vi "Compile Digital Pattern Gen 1.3 Data.vi"(7 "RIO Address":string, 8 "error in (no error)":errorcluster, 11 "Device Item Ref in":T3 format="%.0x") -> (0 "error out":errorcluster, 1 "bitfile names":string[](array[string]), 2 "Digital Pattern Gens":T1[](array[typedef]), 3 "Device Item Ref out":T3 format="%.0x")   [LabVIEW 2017, in "Engine Simulation Toolkit System Explorer.lvlib"]
uses:
  Engine Simulation Toolkit System Explorer.lvlib
  <vilib>/NI Veristand/Custom Device API/Custom Device Item Ref.ctl
  Shared/1.3 Digital Pattern Gen Engine Data.ctl
  Shared/1.3 Digital Pattern Gen FIFO Idxs.ctl
  Digital Pattern Find Events Enum.ctl
  Shared/Constants and GUIDs.vi
  <vilib>/NI Veristand/Custom Device Tools/Custom Device Utility Library/NI VeriStand - Search for Item by GUID.vi
  <vilib>/NI Veristand/Custom Device Tools/Custom Device Utility Library/Custom Device Utility Library.lvlib
  Shared/Engine Simulation Toolkit Shared.lvlib
  <vilib>/NI Veristand/Custom Device API/Custom Device API.lvlib
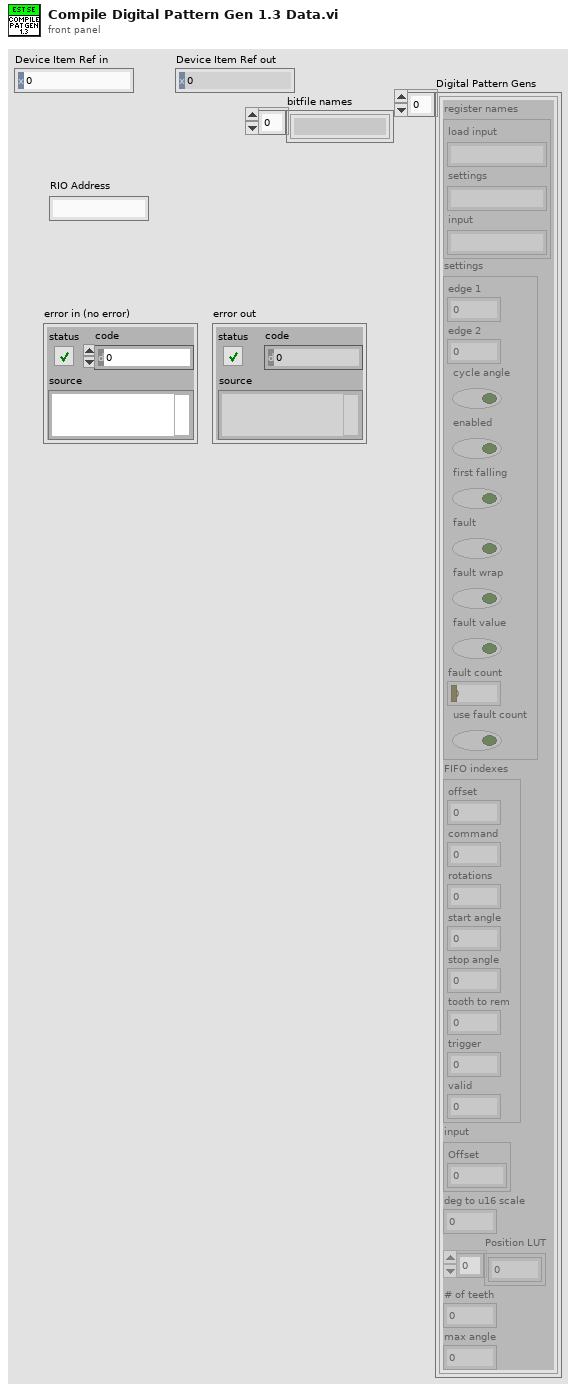
[diagram p1: front panel]
types:
  T1 = typedef "Engine Simulation Toolkit Shared.lvlib/1.3 Digital Pattern Gen Engine Data.ctl" = cluster{"register names":cluster{"load input":string, "settings":string, "input":string}, "settings":cluster{"edge 1":u16, "edge 2":u16, "cycle angle":bool, "enabled":bool, "first falling":bool, "fault":bool, "fault wrap":bool, "fault value":bool, "fault count":fxp<+,4,4>, "use fault count":bool}, "FIFO indexes":T2, "input":cluster{"Offset":i16}, "deg to u16 scale":dbl, "Position LUT":u16[], "# of teeth":i16, "max angle":dbl}
  T2 = typedef "Engine Simulation Toolkit Shared.lvlib/1.3 Digital Pattern Gen FIFO Idxs.ctl" = cluster{"offset":i32, "command":i32, "rotations":i32, "start angle":i32, "stop angle":i32, "tooth to rem":i32, "trigger":i32, "valid":i32}
  T3 = typedef "Custom Device API.lvlib/Custom Device Item Ref.ctl" = u64
  T4 = typedef "Engine Simulation Toolkit Shared.lvlib/Channel.ctl" = cluster{"Name":string, "Units":string, "Default":dbl, "Description":string, "Scalable":bool}
  T5 = typedef "Engine Simulation Toolkit System Explorer.lvlib/Digital Pattern.ctl" = cluster{"Name":string, "Base":T6, "Remove":T7[], "Add":T8[], "FPGA Resource":string}
  T6 = typedef "Engine Simulation Toolkit System Explorer.lvlib/Digital Pattern Base.ctl" = cluster{"Length":dbl, "Teeth":u16, "Width":dbl, "Offset":dbl}
  T7 = typedef "Engine Simulation Toolkit System Explorer.lvlib/Digital Pattern Remove Edge.ctl" = cluster{"Tooth":u16, "Edge":bool}
  T8 = typedef "Engine Simulation Toolkit System Explorer.lvlib/Digital Pattern Add Pulse.ctl" = cluster{"Tooth":u16, "Offset":dbl, "Width":dbl}
  T9 = typedef "Engine Simulation Toolkit System Explorer.lvlib/Digital Pattern Find Events Enum.ctl" = enum16{"Rising Edge", "Falling Edge", "Any Edge", "Center Tooth", "Center Gap"}
  T10 = typedef "Engine Simulation Toolkit System Explorer.lvlib/Digital Pattern Expanded.ctl" = cluster{"X":dbl[], "Y":dbl[]}
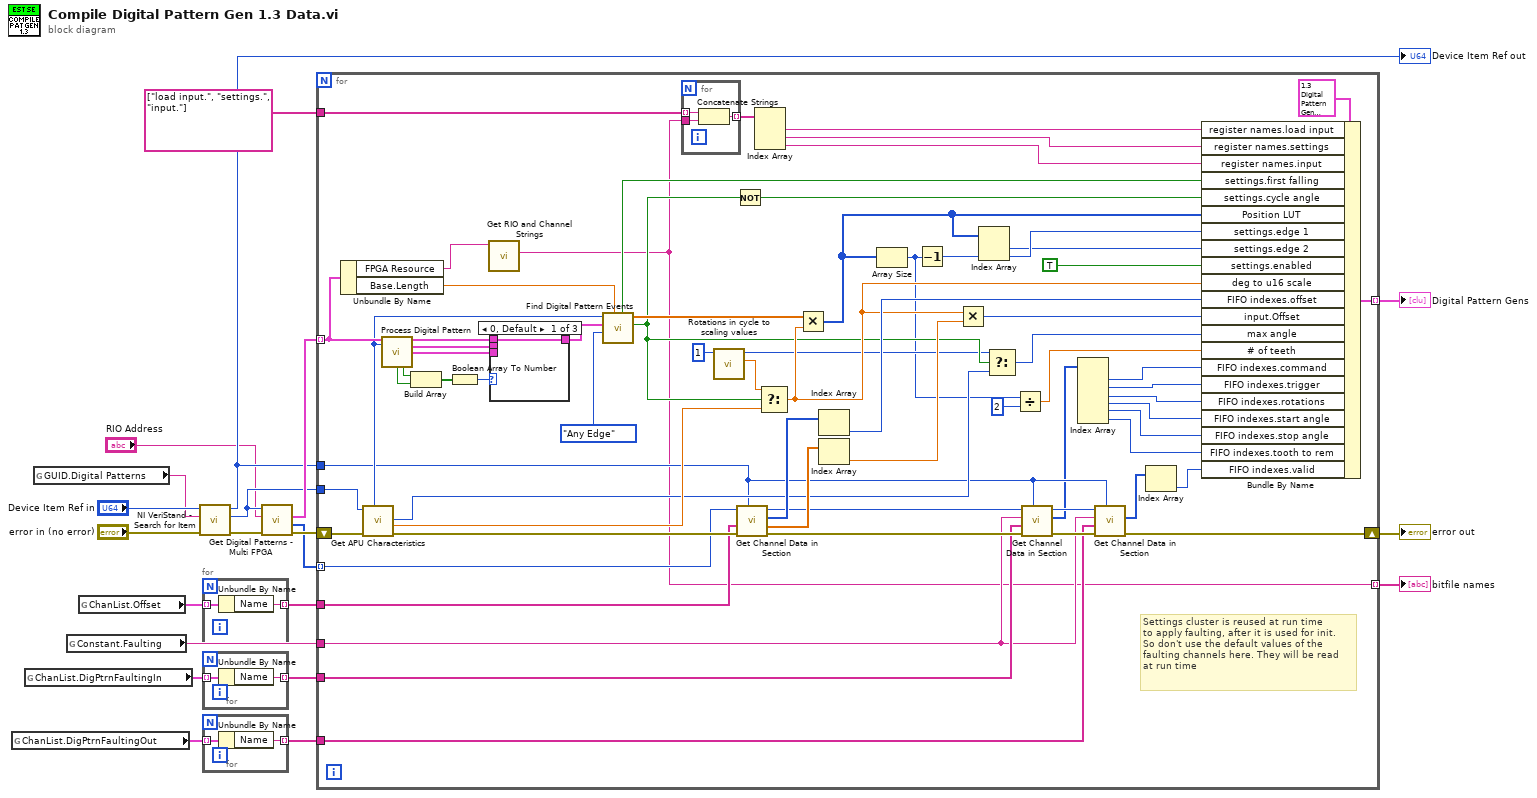
[diagram p0: block diagram]
diagram:
  n1 = global read "Constants and GUIDs.vi" "ChanList.DigPtrnFaultingOut"() -> (w5:T4[])
  n2 = global read "Constants and GUIDs.vi" "ChanList.DigPtrnFaultingIn"() -> (w6:T4[])
  n3 = global read "Constants and GUIDs.vi" "GUID.Digital Patterns"() -> (w19:string)
  n4 = global read "Constants and GUIDs.vi" "Constant.Faulting"() -> (w4:string)
  n5 = global read "Constants and GUIDs.vi" "ChanList.Offset"() -> (w8:T4[])
  n6 = call-poly <vilib>:"NI VeriStand - Search for Item.vi"("error in"="error in (no error)", "Item GUID"=w19, "Section Ref in"="Device Item Ref in") -> ("error out"=w18:errorcluster, "Item Ref"=w10:T3, "Section Ref out"=w11:T3)  [unwired: 5 in, 1 out]
  "Device Item Ref out" <- w11
  n7 = for {
    tunnel: [w23] -> w7 mode=indexing
    tunnel: w8 -> [w22] mode=indexing
    n8 = Unbundle By Name(w22) -> ("Name"=w23:string)
  }
  n9 = for {
    tunnel: [w25] -> w3 mode=indexing
    tunnel: w6 -> [w24] mode=indexing
    n10 = Unbundle By Name(w24) -> ("Name"=w25:string)
  }
  n11 = for {
    tunnel: [w27] -> w2 mode=indexing
    tunnel: w5 -> [w26] mode=indexing
    n12 = Unbundle By Name(w26) -> ("Name"=w27:string)
  }
  n13 = call "Get Digital Patterns - Multi FPGA.vi"("error in (no error)"=w18, "RIO Address"="RIO Address", "Item Ref in"=w10) -> ("error out"=w13:errorcluster, "references"=w9:T3[], "Patterns"=w12:T5[])  [unwired: 6 in]
  n14 = for {
    shift-right: [w30] -> w16
    shift-left: w13 -> [w87]
    tunnel: w12 -> [w85] mode=indexing
    tunnel: string[] ["load input.", "settings.", "input."] -> [w95]
    tunnel: [w90] -> w15 mode=indexing
    tunnel: [w28] -> w14 mode=indexing
    tunnel: w11 -> [w40]
    tunnel: w10 -> [w86]
    tunnel: w9 -> [w74] mode=indexing
    tunnel: w7 -> [w73]
    tunnel: w4 -> [w42]
    tunnel: w3 -> [w43]
    tunnel: w2 -> [w41]
    # "Settings cluster is reused at run time\nto apply faulting, after it is used for init.\nSo don't use the default values of the\nfaulting channels here. They will be read\nat run time"
    n15 = Unbundle By Name(w85) -> ("FPGA Resource"=w29:string, "Base.Length"=w83:dbl)
    n16 = call "Get APU Characteristics.vi"("error in (no error)"=w87, "Item Ref in"=w86) -> ("error out"=w81:errorcluster, "angle to u16 scale factor"=w57:dbl, "total angle span (degrees)"=w52:u16, "rotations"=w84:u16)  [unwired: 3 in, 3 out]
    n17 = call "Process Digital Pattern.vi"("EPT Pattern"=w85, "Rotations"=w84) -> ("Base"=w61:T10, 6:"Reduced"=w60:T10, 8:"Final"=w59:T10, 13:"Final"=w64:bool, 14:"Reduced"=w65:bool)  [unwired: 7 in, 2 out]
    n18 = Build Array(w65, w64) -> (w63:bool[])
    n19 = Boolean Array To Number(Boolean array=w63) -> (number=w62:u32)
    n20 = call "Get RIO and Channel Strings.vi"("rio/channel"=w29) -> ("channel"=w28:string)  [unwired: 9 in, 1 out]
    n21 = case shown="0, Default" w62 {
      tunnel: w61 -> [w96 _ _]
      tunnel: w60 -> [_ w97 _]
      tunnel: w59 -> [_ _ w98]
      tunnel: [w96 w97 w98] -> w58
      frame 0, Default {
      }
      frame 1 {
      }
      frame 2, 3 {
      }
    }
    n22 = call "Find Digital Pattern Events.vi"("Base.length"=w83, "Event"=Digital_Pattern_Find_Events_Enum."Any Edge", "Pattern"=w58, "Rotations"=w84) -> ("crank angle"=w54:bool, "Locations"=w80:dbl[], "first falling"=w55:bool)  [unwired: 5 in]
    n23 = for {
      tunnel: w28 -> [w101]
      tunnel: w95 -> [w100] mode=indexing
      tunnel: [w99] -> w93 mode=indexing
      n24 = Concatenate Strings(w100, w101) -> (w99:string)
    }
    n25 = call "Rotations in cycle to scaling values.vi"("rotations in a cycle"=u16 1) -> ("angle to u16 scale factor"=w56:dbl, "total angle span (degrees)"=w53:u16)  [unwired: 8 in, 1 out]
    n26 = Not(x=w54) -> (.not. x?=w66:bool)
    n27 = call "Get Channel Data in Section.vi"("Custom device ref"=w40, "error in (no error)"=w81, "Channels"=w73, "Item Ref in"=w74) -> ("error out"=w47:errorcluster, "default values"=w70:dbl[], "FIFO indexes"=w72:i32[], "Item Ref out"=w46:T3)  [unwired: 3 in, 1 out]
    n28 = Index Array(array=w93) -> (element #1=w92:string, element #2=w91:string, element #3=w89:string)  [unwired: 3 in]
    n29 = Select(t=w56, s=w54, f=w57) -> (s? t:f=w68:dbl)
    n30 = Multiply(x=w80, y=w68) -> (x*y=w75:u16[])
    n31 = Index Array(array=w72) -> (element=w71:i32)  [unwired: 1 in]
    n32 = Index Array(array=w70) -> (element=w69:dbl)  [unwired: 1 in]
    n33 = Array Size(array=w75) -> (size(s)=w50:i32)
    n34 = Decrement(x=w50) -> (x-1=w78:i32)
    n35 = Multiply(x=w68, y=w69) -> (x*y=w67:i16)
    n36 = Index Array(array=w75, index #2=w78) -> (element #1=w76:u16, element #2=w77:u16)  [unwired: 1 in]
    n37 = Select(t=w53, s=w54, f=w52) -> (s? t:f=w51:u16)
    n38 = Divide(x=w50, y=2) -> (x/y=w48:dbl)
    n39 = call "Get Channel Data in Section.vi"("Custom device ref"=w40, "error in (no error)"=w47, "Channels"=w43, "Section (\"\":none)"=w42, "Item Ref in"=w46) -> ("error out"=w45:errorcluster, "FIFO indexes"=w39:i32[], "Item Ref out"=w44:T3)  [unwired: 2 in, 2 out]
    n40 = Index Array(array=w39) -> (element #1=w38:i32, element #2=w37:i32, element #3=w36:i32, element #4=w35:i32, element #5=w34:i32, element #6=w33:i32)  [unwired: 6 in]
    n41 = call "Get Channel Data in Section.vi"("Custom device ref"=w40, "error in (no error)"=w45, "Channels"=w41, "Section (\"\":none)"=w42, "Item Ref in"=w44) -> ("error out"=w30:errorcluster, "FIFO indexes"=w32:i32[])  [unwired: 2 in, 3 out]
    n42 = Index Array(array=w32) -> (element=w31:i32)  [unwired: 1 in]
    n43 = Bundle By Name(cluster=T1 {"register names"={"load input"="", "settings"="", "input"=""}, "settings"={"edge 1"=0, "edge 2"=0, "cycle angle"=FALSE, "enabled"=FALSE, "first falling"=FALSE, "fault"=FALSE, "fault wrap"=FALSE, "fault value"=FALSE, "fault count"=0.0, "use fault count"=FALSE}, "FIFO indexes"={"offset"=0, "command"=0, "rotations"=0, "start angle"=0, "stop angle"=0, "tooth to rem"=0, "trigger"=0, "valid"=0}, "input"={"Offset"=0}, "deg to u16 scale"=0.0, "Position LUT"=[], "# of teeth"=0, "max angle"=0.0} ("1.0.0 Digital Pattern Gen"), "register names.load input"=w92, "register names.settings"=w91, "register names.input"=w89, "settings.first falling"=w55, "settings.cycle angle"=w66, "Position LUT"=w75, "settings.edge 1"=w77, "settings.edge 2"=w76, "settings.enabled"=TRUE, "deg to u16 scale"=w68, "FIFO indexes.offset"=w71, "input.Offset"=w67, "max angle"=w51, "# of teeth"=w48, "FIFO indexes.command"=w38, "FIFO indexes.trigger"=w37, "FIFO indexes.rotations"=w36, "FIFO indexes.start angle"=w35, "FIFO indexes.stop angle"=w34, "FIFO indexes.tooth to rem"=w33, "FIFO indexes.valid"=w31) -> (w90:T1)
  }
  "error out" <- w16
  "Digital Pattern Gens" <- w15
  "bitfile names" <- w14
